vi "WILT Step 6.vi"(7 "Station Number in":u32, 8 "Error In":errorcluster, 10 "Step 3 Input":T1, 11 "Dryer Step 5 In":T3 {"Night Cycle Count" format="%04d"; "Day Cycle Count" format="%04d"}) -> (0 "Error Out":errorcluster, 2 "Step 5 Output":T1, 3 "Dryer Step 5 Output":T3 {"Night Cycle Count" format="%04d"; "Day Cycle Count" format="%04d"})   [LabVIEW 2016]
uses:
  Type Definitions/WILT Station Test State Cluster.ctl
  Type Definitions/WILT Dryer Test State.ctl
  Type Definitions/WILT Dryer.ctl
  Type Definitions/WILT Dryer Details.ctl
  Type Definitions/WILT Agilent Channel Definition.ctl
  Type Definitions/WILT DAQ Data.ctl
  Globals/WILT Globals Main Program.vi
panel:
  # "Day"
  # "Night"
  # "Day"
  # "Night"
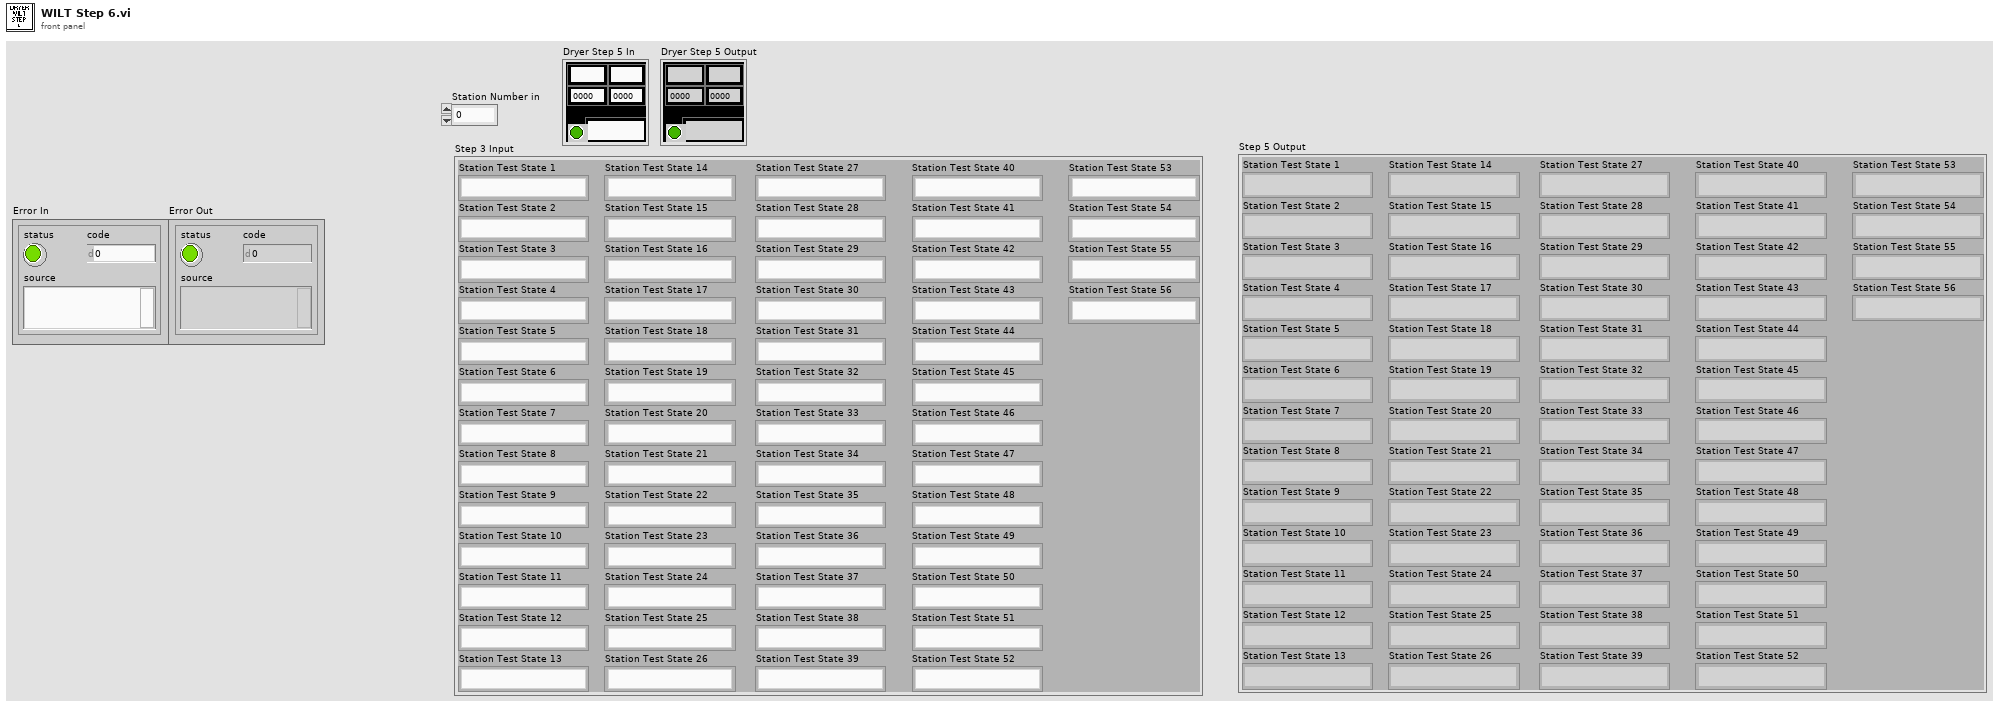
[diagram p1: front panel]
types:
  T1 = typedef "WILT Station Test State Cluster.ctl" = cluster{"Station Test State 1":T2, "Station Test State 2":T2, "Station Test State 3":T2, "Station Test State 4":T2, "Station Test State 5":T2, "Station Test State 6":T2, "Station Test State 7":T2, "Station Test State 8":T2, "Station Test State 9":T2, "Station Test State 10":T2, "Station Test State 11":T2, "Station Test State 12":T2, "Station Test State 13":T2, "Station Test State 14":T2, "Station Test State 15":T2, "Station Test State 16":T2, "Station Test State 17":T2, "Station Test State 18":T2, "Station Test State 19":T2, "Station Test State 20":T2, "Station Test State 21":T2, "Station Test State 22":T2, "Station Test State 23":T2, "Station Test State 24":T2, "Station Test State 25":T2, "Station Test State 26":T2, "Station Test State 27":T2, "Station Test State 28":T2, "Station Test State 29":T2, "Station Test State 30":T2, "Station Test State 31":T2, "Station Test State 32":T2, "Station Test State 33":T2, "Station Test State 34":T2, "Station Test State 35":T2, "Station Test State 36":T2, "Station Test State 37":T2, "Station Test State 38":T2, "Station Test State 39":T2, "Station Test State 40":T2, "Station Test State 41":T2, "Station Test State 42":T2, "Station Test State 43":T2, "Station Test State 44":T2, "Station Test State 45":T2, "Station Test State 46":T2, "Station Test State 47":T2, "Station Test State 48":T2, "Station Test State 49":T2, "Station Test State 50":T2, "Station Test State 51":T2, "Station Test State 52":T2, "Station Test State 53":T2, "Station Test State 54":T2, "Station Test State 55":T2, "Station Test State 56":T2}
  T2 = typedef "WILT Dryer Test State.ctl" = enum16{"No Serial Number", "Waiting for Dryer To Start", "Drying Clothes", "Water Injection 1 (On)", "Water Injection 1 Timer", "Water Injection 1 (Off)", "Pause Dryer", "Sending Start Stop CMD", "Pause Dryer 2", "Sending Start Stop CMD 2", "Drying Clothes 2", "Water Injection 2 (On)", "Water Injection 2 Timer", "Water Injection 2 (Off)", "Drying Clothes 3", "Cooling Down", "Sending Start Stop CMD 3", "Increment Cycle"}
  T3 = typedef "WILT Dryer.ctl" = cluster{"Lab ID":string, "Day Cycle Count":i32, "Station Label":string, "Dryer Details":T4, "Status Color":u32, "Invisible Button":bool, "Night Cycle Count":i32, "Station Index":i32, "Cycle Index":string, "Audit Alert":bool, "Agilent Channel Definition":T5, "DAQ Data":T6}
  T4 = typedef "WILT Dryer Details.ctl" = cluster{"Station":string, "Lab ID":string, "TR Number":string}
  T5 = typedef "WILT Agilent Channel Definition.ctl" = cluster{"Channel":string, "Station":string, "Label":string, "Agilent Station":string, "Data":dbl}
  T6 = typedef "WILT DAQ Data.ctl" = cluster{"L1 Current":dbl, "L2 Current":dbl, "Temperature  Deg F (TC)":dbl, "Volts":dbl, "Volts (208)":dbl, "SW (208)":dbl}
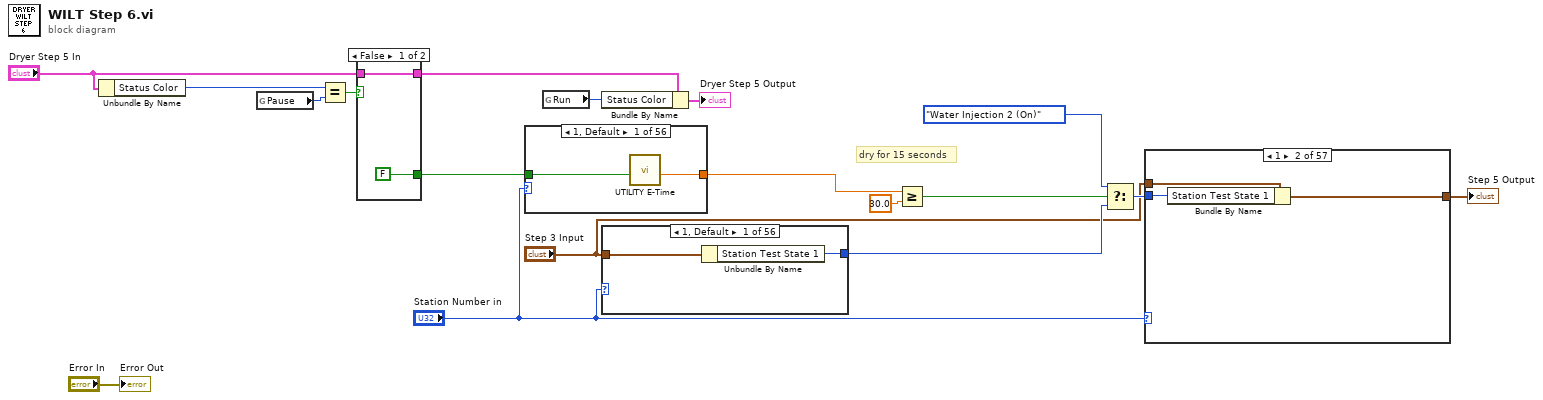
[diagram p0: block diagram]
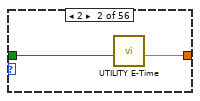
[diagram p2: hidden frame]
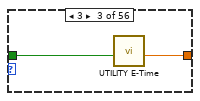
[diagram p3: hidden frame]
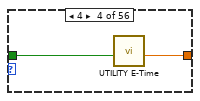
[diagram p4: hidden frame]
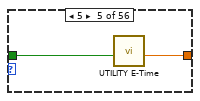
[diagram p5: hidden frame]
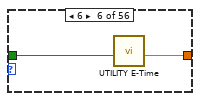
[diagram p6: hidden frame]
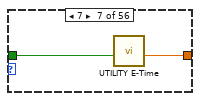
[diagram p7: hidden frame]
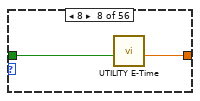
[diagram p8: hidden frame]
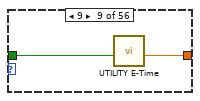
[diagram p9: hidden frame]
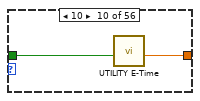
[diagram p10: hidden frame]
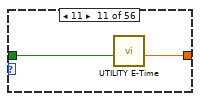
[diagram p11: hidden frame]
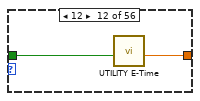
[diagram p12: hidden frame]
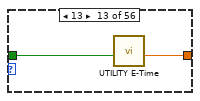
[diagram p13: hidden frame]
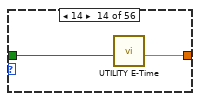
[diagram p14: hidden frame]
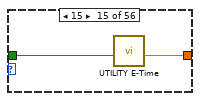
[diagram p15: hidden frame]
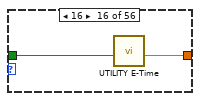
[diagram p16: hidden frame]
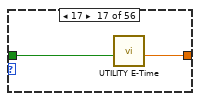
[diagram p17: hidden frame]
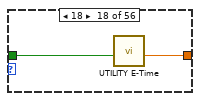
[diagram p18: hidden frame]
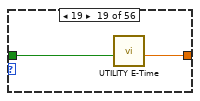
[diagram p19: hidden frame]
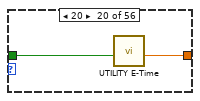
[diagram p20: hidden frame]
diagram:
  # "dry for 15 seconds"
  n1 = Unbundle By Name("Dryer Step 5 In") -> ("Status Color"=w12:u32)
  n2 = global read "WILT Globals Main Program.vi" "Pause"() -> (w4:u32)
  n3 = Equal?(x=w12, y=w4) -> (x = y?=w5:bool)
  n4 = case shown="False" w5 {
    tunnel: [FALSE TRUE] -> w2
    tunnel: "Dryer Step 5 In" -> [w19 w21]
    tunnel: [w19 w21] -> w3
    frame False {
    }
    frame True {
    }
  }
  n5 = case shown="1, Default" "Station Number in" {
    tunnel: [w24 w25 w27 w29 w31 w33 w35 w37 w39 w41 w43 w45 w47 w49 w51 w53 w55 w57 w59 w61 w63 w65 w67 w69 w71 w73 w75 w77 w79 w81 w83 w85 w87 w89 w91 w93 w95 w97 w99 w101 w103 w105 w107 w109 w111 w113 w115 w117 w119 w121 w123 w125 w127 w129 w131 w133] -> w1
    tunnel: w2 -> [w23 w26 w28 w30 w32 w34 w36 w38 w40 w42 w44 w46 w48 w50 w52 w54 w56 w58 w60 w62 w64 w66 w68 w70 w72 w74 w76 w78 w80 w82 w84 w86 w88 w90 w92 w94 w96 w98 w100 w102 w104 w106 w108 w110 w112 w114 w116 w118 w120 w122 w124 w126 w128 w130 w132 w134]
    frame 1, Default {
      n6 = call "UTILITY E-Time.vi"("Reset"=w23) -> ("Elapsed Time (sec)"=w24:dbl)  [unwired: 8 in, 2 out]
    }
    frame 2 {
      n7 = call "UTILITY E-Time.vi"("Reset"=w26) -> ("Elapsed Time (sec)"=w25:dbl)  [unwired: 8 in, 2 out]
    }
    frame 3 {
      n8 = call "UTILITY E-Time.vi"("Reset"=w28) -> ("Elapsed Time (sec)"=w27:dbl)  [unwired: 8 in, 2 out]
    }
    frame 4 {
      n9 = call "UTILITY E-Time.vi"("Reset"=w30) -> ("Elapsed Time (sec)"=w29:dbl)  [unwired: 8 in, 2 out]
    }
    frame 5 {
      n10 = call "UTILITY E-Time.vi"("Reset"=w32) -> ("Elapsed Time (sec)"=w31:dbl)  [unwired: 8 in, 2 out]
    }
    frame 6 {
      n11 = call "UTILITY E-Time.vi"("Reset"=w34) -> ("Elapsed Time (sec)"=w33:dbl)  [unwired: 8 in, 2 out]
    }
    frame 7 {
      n12 = call "UTILITY E-Time.vi"("Reset"=w36) -> ("Elapsed Time (sec)"=w35:dbl)  [unwired: 8 in, 2 out]
    }
    frame 8 {
      n13 = call "UTILITY E-Time.vi"("Reset"=w38) -> ("Elapsed Time (sec)"=w37:dbl)  [unwired: 8 in, 2 out]
    }
    frame 9 {
      n14 = call "UTILITY E-Time.vi"("Reset"=w40) -> ("Elapsed Time (sec)"=w39:dbl)  [unwired: 8 in, 2 out]
    }
    frame 10 {
      n15 = call "UTILITY E-Time.vi"("Reset"=w42) -> ("Elapsed Time (sec)"=w41:dbl)  [unwired: 8 in, 2 out]
    }
    frame 11 {
      n16 = call "UTILITY E-Time.vi"("Reset"=w44) -> ("Elapsed Time (sec)"=w43:dbl)  [unwired: 8 in, 2 out]
    }
    frame 12 {
      n17 = call "UTILITY E-Time.vi"("Reset"=w46) -> ("Elapsed Time (sec)"=w45:dbl)  [unwired: 8 in, 2 out]
    }
    frame 13 {
      n18 = call "UTILITY E-Time.vi"("Reset"=w48) -> ("Elapsed Time (sec)"=w47:dbl)  [unwired: 8 in, 2 out]
    }
    frame 14 {
      n19 = call "UTILITY E-Time.vi"("Reset"=w50) -> ("Elapsed Time (sec)"=w49:dbl)  [unwired: 8 in, 2 out]
    }
    frame 15 {
      n20 = call "UTILITY E-Time.vi"("Reset"=w52) -> ("Elapsed Time (sec)"=w51:dbl)  [unwired: 8 in, 2 out]
    }
    frame 16 {
      n21 = call "UTILITY E-Time.vi"("Reset"=w54) -> ("Elapsed Time (sec)"=w53:dbl)  [unwired: 8 in, 2 out]
    }
    frame 17 {
      n22 = call "UTILITY E-Time.vi"("Reset"=w56) -> ("Elapsed Time (sec)"=w55:dbl)  [unwired: 8 in, 2 out]
    }
    frame 18 {
      n23 = call "UTILITY E-Time.vi"("Reset"=w58) -> ("Elapsed Time (sec)"=w57:dbl)  [unwired: 8 in, 2 out]
    }
    frame 19 {
      n24 = call "UTILITY E-Time.vi"("Reset"=w60) -> ("Elapsed Time (sec)"=w59:dbl)  [unwired: 8 in, 2 out]
    }
    frame 20 {
      n25 = call "UTILITY E-Time.vi"("Reset"=w62) -> ("Elapsed Time (sec)"=w61:dbl)  [unwired: 8 in, 2 out]
    }
    frame 21 {
      n26 = call "UTILITY E-Time.vi"("Reset"=w64) -> ("Elapsed Time (sec)"=w63:dbl)  [unwired: 8 in, 2 out]
    }
    frame 22 {
      n27 = call "UTILITY E-Time.vi"("Reset"=w66) -> ("Elapsed Time (sec)"=w65:dbl)  [unwired: 8 in, 2 out]
    }
    frame 23 {
      n28 = call "UTILITY E-Time.vi"("Reset"=w68) -> ("Elapsed Time (sec)"=w67:dbl)  [unwired: 8 in, 2 out]
    }
    frame 24 {
      n29 = call "UTILITY E-Time.vi"("Reset"=w70) -> ("Elapsed Time (sec)"=w69:dbl)  [unwired: 8 in, 2 out]
    }
    frame 25 {
      n30 = call "UTILITY E-Time.vi"("Reset"=w72) -> ("Elapsed Time (sec)"=w71:dbl)  [unwired: 8 in, 2 out]
    }
    frame 26 {
      n31 = call "UTILITY E-Time.vi"("Reset"=w74) -> ("Elapsed Time (sec)"=w73:dbl)  [unwired: 8 in, 2 out]
    }
    frame 27 {
      n32 = call "UTILITY E-Time.vi"("Reset"=w76) -> ("Elapsed Time (sec)"=w75:dbl)  [unwired: 8 in, 2 out]
    }
    frame 28 {
      n33 = call "UTILITY E-Time.vi"("Reset"=w78) -> ("Elapsed Time (sec)"=w77:dbl)  [unwired: 8 in, 2 out]
    }
    frame 29 {
      n34 = call "UTILITY E-Time.vi"("Reset"=w80) -> ("Elapsed Time (sec)"=w79:dbl)  [unwired: 8 in, 2 out]
    }
    frame 30 {
      n35 = call "UTILITY E-Time.vi"("Reset"=w82) -> ("Elapsed Time (sec)"=w81:dbl)  [unwired: 8 in, 2 out]
    }
    frame 31 {
      n36 = call "UTILITY E-Time.vi"("Reset"=w84) -> ("Elapsed Time (sec)"=w83:dbl)  [unwired: 8 in, 2 out]
    }
    frame 32 {
      n37 = call "UTILITY E-Time.vi"("Reset"=w86) -> ("Elapsed Time (sec)"=w85:dbl)  [unwired: 8 in, 2 out]
    }
    frame 33 {
      n38 = call "UTILITY E-Time.vi"("Reset"=w88) -> ("Elapsed Time (sec)"=w87:dbl)  [unwired: 8 in, 2 out]
    }
    frame 34 {
      n39 = call "UTILITY E-Time.vi"("Reset"=w90) -> ("Elapsed Time (sec)"=w89:dbl)  [unwired: 8 in, 2 out]
    }
    frame 35 {
      n40 = call "UTILITY E-Time.vi"("Reset"=w92) -> ("Elapsed Time (sec)"=w91:dbl)  [unwired: 8 in, 2 out]
    }
    frame 36 {
      n41 = call "UTILITY E-Time.vi"("Reset"=w94) -> ("Elapsed Time (sec)"=w93:dbl)  [unwired: 8 in, 2 out]
    }
    frame 37 {
      n42 = call "UTILITY E-Time.vi"("Reset"=w96) -> ("Elapsed Time (sec)"=w95:dbl)  [unwired: 8 in, 2 out]
    }
    frame 38 {
      n43 = call "UTILITY E-Time.vi"("Reset"=w98) -> ("Elapsed Time (sec)"=w97:dbl)  [unwired: 8 in, 2 out]
    }
    frame 39 {
      n44 = call "UTILITY E-Time.vi"("Reset"=w100) -> ("Elapsed Time (sec)"=w99:dbl)  [unwired: 8 in, 2 out]
    }
    frame 40 {
      n45 = call "UTILITY E-Time.vi"("Reset"=w102) -> ("Elapsed Time (sec)"=w101:dbl)  [unwired: 8 in, 2 out]
    }
    frame 41 {
      n46 = call "UTILITY E-Time.vi"("Reset"=w104) -> ("Elapsed Time (sec)"=w103:dbl)  [unwired: 8 in, 2 out]
    }
    frame 42 {
      n47 = call "UTILITY E-Time.vi"("Reset"=w106) -> ("Elapsed Time (sec)"=w105:dbl)  [unwired: 8 in, 2 out]
    }
    frame 43 {
      n48 = call "UTILITY E-Time.vi"("Reset"=w108) -> ("Elapsed Time (sec)"=w107:dbl)  [unwired: 8 in, 2 out]
    }
    frame 44 {
      n49 = call "UTILITY E-Time.vi"("Reset"=w110) -> ("Elapsed Time (sec)"=w109:dbl)  [unwired: 8 in, 2 out]
    }
    frame 45 {
      n50 = call "UTILITY E-Time.vi"("Reset"=w112) -> ("Elapsed Time (sec)"=w111:dbl)  [unwired: 8 in, 2 out]
    }
    frame 46 {
      n51 = call "UTILITY E-Time.vi"("Reset"=w114) -> ("Elapsed Time (sec)"=w113:dbl)  [unwired: 8 in, 2 out]
    }
    frame 47 {
      n52 = call "UTILITY E-Time.vi"("Reset"=w116) -> ("Elapsed Time (sec)"=w115:dbl)  [unwired: 8 in, 2 out]
    }
    frame 48 {
      n53 = call "UTILITY E-Time.vi"("Reset"=w118) -> ("Elapsed Time (sec)"=w117:dbl)  [unwired: 8 in, 2 out]
    }
    frame 49 {
      n54 = call "UTILITY E-Time.vi"("Reset"=w120) -> ("Elapsed Time (sec)"=w119:dbl)  [unwired: 8 in, 2 out]
    }
    frame 50 {
      n55 = call "UTILITY E-Time.vi"("Reset"=w122) -> ("Elapsed Time (sec)"=w121:dbl)  [unwired: 8 in, 2 out]
    }
    frame 51 {
      n56 = call "UTILITY E-Time.vi"("Reset"=w124) -> ("Elapsed Time (sec)"=w123:dbl)  [unwired: 8 in, 2 out]
    }
    frame 52 {
      n57 = call "UTILITY E-Time.vi"("Reset"=w126) -> ("Elapsed Time (sec)"=w125:dbl)  [unwired: 8 in, 2 out]
    }
    frame 53 {
      n58 = call "UTILITY E-Time.vi"("Reset"=w128) -> ("Elapsed Time (sec)"=w127:dbl)  [unwired: 8 in, 2 out]
    }
    frame 54 {
      n59 = call "UTILITY E-Time.vi"("Reset"=w130) -> ("Elapsed Time (sec)"=w129:dbl)  [unwired: 8 in, 2 out]
    }
    frame 55 {
      n60 = call "UTILITY E-Time.vi"("Reset"=w132) -> ("Elapsed Time (sec)"=w131:dbl)  [unwired: 8 in, 2 out]
    }
    frame 56 {
      n61 = call "UTILITY E-Time.vi"("Reset"=w134) -> ("Elapsed Time (sec)"=w133:dbl)  [unwired: 8 in, 2 out]
    }
  }
  n62 = global read "WILT Globals Main Program.vi" "Run"() -> (w6:u32)
  n63 = Bundle By Name(cluster=w3, "Status Color"=w6) -> (→"Dryer Step 5 Output":T3)
  n64 = case shown="1, Default" "Station Number in" {
    tunnel: "Step 3 Input" -> [w136 w138 w140 w142 w144 w146 w148 w150 w152 w154 w156 w158 w160 w162 w164 w166 w168 w170 w172 w174 w176 w178 w180 w182 w184 w186 w188 w190 w192 w194 w196 w198 w200 w202 w204 w206 w208 w210 w212 w214 w216 w218 w220 w222 w224 w226 w228 w230 w232 w234 w236 w238 w240 w242 w244 w246]
    tunnel: [w135 w137 w139 w141 w143 w145 w147 w149 w151 w153 w155 w157 w159 w161 w163 w165 w167 w169 w171 w173 w175 w177 w179 w181 w183 w185 w187 w189 w191 w193 w195 w197 w199 w201 w203 w205 w207 w209 w211 w213 w215 w217 w219 w221 w223 w225 w227 w229 w231 w233 w235 w237 w239 w241 w243 w245] -> w17
    frame 1, Default {
      n65 = Unbundle By Name(w136) -> ("Station Test State 1"=w135:T2)
    }
    frame 2 {
      n66 = Unbundle By Name(w138) -> ("Station Test State 2"=w137:T2)
    }
    frame 3 {
      n67 = Unbundle By Name(w140) -> ("Station Test State 3"=w139:T2)
    }
    frame 4 {
      n68 = Unbundle By Name(w142) -> ("Station Test State 4"=w141:T2)
    }
    frame 5 {
      n69 = Unbundle By Name(w144) -> ("Station Test State 5"=w143:T2)
    }
    frame 6 {
      n70 = Unbundle By Name(w146) -> ("Station Test State 6"=w145:T2)
    }
    frame 7 {
      n71 = Unbundle By Name(w148) -> ("Station Test State 7"=w147:T2)
    }
    frame 8 {
      n72 = Unbundle By Name(w150) -> ("Station Test State 8"=w149:T2)
    }
    frame 9 {
      n73 = Unbundle By Name(w152) -> ("Station Test State 9"=w151:T2)
    }
    frame 10 {
      n74 = Unbundle By Name(w154) -> ("Station Test State 10"=w153:T2)
    }
    frame 11 {
      n75 = Unbundle By Name(w156) -> ("Station Test State 11"=w155:T2)
    }
    frame 12 {
      n76 = Unbundle By Name(w158) -> ("Station Test State 12"=w157:T2)
    }
    frame 13 {
      n77 = Unbundle By Name(w160) -> ("Station Test State 13"=w159:T2)
    }
    frame 14 {
      n78 = Unbundle By Name(w162) -> ("Station Test State 14"=w161:T2)
    }
    frame 15 {
      n79 = Unbundle By Name(w164) -> ("Station Test State 15"=w163:T2)
    }
    frame 16 {
      n80 = Unbundle By Name(w166) -> ("Station Test State 16"=w165:T2)
    }
    frame 17 {
      n81 = Unbundle By Name(w168) -> ("Station Test State 17"=w167:T2)
    }
    frame 18 {
      n82 = Unbundle By Name(w170) -> ("Station Test State 18"=w169:T2)
    }
    frame 19 {
      n83 = Unbundle By Name(w172) -> ("Station Test State 19"=w171:T2)
    }
    frame 20 {
      n84 = Unbundle By Name(w174) -> ("Station Test State 20"=w173:T2)
    }
    frame 21 {
      n85 = Unbundle By Name(w176) -> ("Station Test State 21"=w175:T2)
    }
    frame 22 {
      n86 = Unbundle By Name(w178) -> ("Station Test State 22"=w177:T2)
    }
    frame 23 {
      n87 = Unbundle By Name(w180) -> ("Station Test State 23"=w179:T2)
    }
    frame 24 {
      n88 = Unbundle By Name(w182) -> ("Station Test State 24"=w181:T2)
    }
    frame 25 {
      n89 = Unbundle By Name(w184) -> ("Station Test State 25"=w183:T2)
    }
    frame 26 {
      n90 = Unbundle By Name(w186) -> ("Station Test State 26"=w185:T2)
    }
    frame 27 {
      n91 = Unbundle By Name(w188) -> ("Station Test State 27"=w187:T2)
    }
    frame 28 {
      n92 = Unbundle By Name(w190) -> ("Station Test State 28"=w189:T2)
    }
    frame 29 {
      n93 = Unbundle By Name(w192) -> ("Station Test State 29"=w191:T2)
    }
    frame 30 {
      n94 = Unbundle By Name(w194) -> ("Station Test State 30"=w193:T2)
    }
    frame 31 {
      n95 = Unbundle By Name(w196) -> ("Station Test State 31"=w195:T2)
    }
    frame 32 {
      n96 = Unbundle By Name(w198) -> ("Station Test State 32"=w197:T2)
    }
    frame 33 {
      n97 = Unbundle By Name(w200) -> ("Station Test State 33"=w199:T2)
    }
    frame 34 {
      n98 = Unbundle By Name(w202) -> ("Station Test State 34"=w201:T2)
    }
    frame 35 {
      n99 = Unbundle By Name(w204) -> ("Station Test State 35"=w203:T2)
    }
    frame 36 {
      n100 = Unbundle By Name(w206) -> ("Station Test State 36"=w205:T2)
    }
    frame 37 {
      n101 = Unbundle By Name(w208) -> ("Station Test State 37"=w207:T2)
    }
    frame 38 {
      n102 = Unbundle By Name(w210) -> ("Station Test State 38"=w209:T2)
    }
    frame 39 {
      n103 = Unbundle By Name(w212) -> ("Station Test State 39"=w211:T2)
    }
    frame 40 {
      n104 = Unbundle By Name(w214) -> ("Station Test State 40"=w213:T2)
    }
    frame 41 {
      n105 = Unbundle By Name(w216) -> ("Station Test State 41"=w215:T2)
    }
    frame 42 {
      n106 = Unbundle By Name(w218) -> ("Station Test State 42"=w217:T2)
    }
    frame 43 {
      n107 = Unbundle By Name(w220) -> ("Station Test State 43"=w219:T2)
    }
    frame 44 {
      n108 = Unbundle By Name(w222) -> ("Station Test State 44"=w221:T2)
    }
    frame 45 {
      n109 = Unbundle By Name(w224) -> ("Station Test State 45"=w223:T2)
    }
    frame 46 {
      n110 = Unbundle By Name(w226) -> ("Station Test State 46"=w225:T2)
    }
    frame 47 {
      n111 = Unbundle By Name(w228) -> ("Station Test State 47"=w227:T2)
    }
    frame 48 {
      n112 = Unbundle By Name(w230) -> ("Station Test State 48"=w229:T2)
    }
    frame 49 {
      n113 = Unbundle By Name(w232) -> ("Station Test State 49"=w231:T2)
    }
    frame 50 {
      n114 = Unbundle By Name(w234) -> ("Station Test State 50"=w233:T2)
    }
    frame 51 {
      n115 = Unbundle By Name(w236) -> ("Station Test State 51"=w235:T2)
    }
    frame 52 {
      n116 = Unbundle By Name(w238) -> ("Station Test State 52"=w237:T2)
    }
    frame 53 {
      n117 = Unbundle By Name(w240) -> ("Station Test State 53"=w239:T2)
    }
    frame 54 {
      n118 = Unbundle By Name(w242) -> ("Station Test State 54"=w241:T2)
    }
    frame 55 {
      n119 = Unbundle By Name(w244) -> ("Station Test State 55"=w243:T2)
    }
    frame 56 {
      n120 = Unbundle By Name(w246) -> ("Station Test State 56"=w245:T2)
    }
  }
  n121 = Greater Or Equal?(x=w1, y=30.0) -> (x >= y?=w14:bool)
  n122 = Select(t=WILT_Dryer_Test_State."Water Injection 2 (On)" ("Current State 2"), s=w14, f=w17) -> (s? t:f=w18:T2)
  n123 = case shown="1" "Station Number in" {
    tunnel: "Step 3 Input" -> [w247 w250 w253 w256 w259 w262 w265 w268 w271 w274 w277 w280 w283 w286 w289 w292 w295 w298 w301 w304 w307 w310 w313 w316 w319 w322 w325 w328 w331 w334 w337 w340 w343 w346 w349 w352 w355 w358 w361 w364 w367 w370 w373 w376 w379 w382 w385 w388 w391 w394 w397 w400 w403 w406 w409 w412 w415]
    tunnel: w18 -> [_ w249 w251 w254 w257 w260 w263 w266 w269 w272 w275 w278 w281 w284 w287 w290 w293 w296 w299 w302 w305 w308 w311 w314 w317 w320 w323 w326 w329 w332 w335 w338 w341 w344 w347 w350 w353 w356 w359 w362 w365 w368 w371 w374 w377 w380 w383 w386 w389 w392 w395 w398 w401 w404 w407 w410 w413]
    tunnel: [w247 w248 w252 w255 w258 w261 w264 w267 w270 w273 w276 w279 w282 w285 w288 w291 w294 w297 w300 w303 w306 w309 w312 w315 w318 w321 w324 w327 w330 w333 w336 w339 w342 w345 w348 w351 w354 w357 w360 w363 w366 w369 w372 w375 w378 w381 w384 w387 w390 w393 w396 w399 w402 w405 w408 w411 w414] -> w15
    frame 0, Default {
      # "Not a valid station. Do nothing"
    }
    frame 1 {
      n124 = Bundle By Name(cluster=w250, "Station Test State 1"=w249) -> (w248:T1)
    }
    frame 2 {
      n125 = Bundle By Name(cluster=w253, "Station Test State 2"=w251) -> (w252:T1)
    }
    frame 3 {
      n126 = Bundle By Name(cluster=w256, "Station Test State 3"=w254) -> (w255:T1)
    }
    frame 4 {
      n127 = Bundle By Name(cluster=w259, "Station Test State 4"=w257) -> (w258:T1)
    }
    frame 5 {
      n128 = Bundle By Name(cluster=w262, "Station Test State 5"=w260) -> (w261:T1)
    }
    frame 6 {
      n129 = Bundle By Name(cluster=w265, "Station Test State 6"=w263) -> (w264:T1)
    }
    frame 7 {
      n130 = Bundle By Name(cluster=w268, "Station Test State 7"=w266) -> (w267:T1)
    }
    frame 8 {
      n131 = Bundle By Name(cluster=w271, "Station Test State 8"=w269) -> (w270:T1)
    }
    frame 9 {
      n132 = Bundle By Name(cluster=w274, "Station Test State 9"=w272) -> (w273:T1)
    }
    frame 10 {
      n133 = Bundle By Name(cluster=w277, "Station Test State 10"=w275) -> (w276:T1)
    }
    frame 11 {
      n134 = Bundle By Name(cluster=w280, "Station Test State 11"=w278) -> (w279:T1)
    }
    frame 12 {
      n135 = Bundle By Name(cluster=w283, "Station Test State 12"=w281) -> (w282:T1)
    }
    frame 13 {
      n136 = Bundle By Name(cluster=w286, "Station Test State 13"=w284) -> (w285:T1)
    }
    frame 14 {
      n137 = Bundle By Name(cluster=w289, "Station Test State 14"=w287) -> (w288:T1)
    }
    frame 15 {
      n138 = Bundle By Name(cluster=w292, "Station Test State 15"=w290) -> (w291:T1)
    }
    frame 16 {
      n139 = Bundle By Name(cluster=w295, "Station Test State 16"=w293) -> (w294:T1)
    }
    frame 17 {
      n140 = Bundle By Name(cluster=w298, "Station Test State 17"=w296) -> (w297:T1)
    }
    frame 18 {
      n141 = Bundle By Name(cluster=w301, "Station Test State 18"=w299) -> (w300:T1)
    }
    frame 19 {
      n142 = Bundle By Name(cluster=w304, "Station Test State 19"=w302) -> (w303:T1)
    }
    frame 20 {
      n143 = Bundle By Name(cluster=w307, "Station Test State 20"=w305) -> (w306:T1)
    }
    frame 21 {
      n144 = Bundle By Name(cluster=w310, "Station Test State 21"=w308) -> (w309:T1)
    }
    frame 22 {
      n145 = Bundle By Name(cluster=w313, "Station Test State 22"=w311) -> (w312:T1)
    }
    frame 23 {
      n146 = Bundle By Name(cluster=w316, "Station Test State 23"=w314) -> (w315:T1)
    }
    frame 24 {
      n147 = Bundle By Name(cluster=w319, "Station Test State 24"=w317) -> (w318:T1)
    }
    frame 25 {
      n148 = Bundle By Name(cluster=w322, "Station Test State 25"=w320) -> (w321:T1)
    }
    frame 26 {
      n149 = Bundle By Name(cluster=w325, "Station Test State 26"=w323) -> (w324:T1)
    }
    frame 27 {
      n150 = Bundle By Name(cluster=w328, "Station Test State 27"=w326) -> (w327:T1)
    }
    frame 28 {
      n151 = Bundle By Name(cluster=w331, "Station Test State 28"=w329) -> (w330:T1)
    }
    frame 29 {
      n152 = Bundle By Name(cluster=w334, "Station Test State 29"=w332) -> (w333:T1)
    }
    frame 30 {
      n153 = Bundle By Name(cluster=w337, "Station Test State 30"=w335) -> (w336:T1)
    }
    frame 31 {
      n154 = Bundle By Name(cluster=w340, "Station Test State 31"=w338) -> (w339:T1)
    }
    frame 32 {
      n155 = Bundle By Name(cluster=w343, "Station Test State 32"=w341) -> (w342:T1)
    }
    frame 33 {
      n156 = Bundle By Name(cluster=w346, "Station Test State 33"=w344) -> (w345:T1)
    }
    frame 34 {
      n157 = Bundle By Name(cluster=w349, "Station Test State 34"=w347) -> (w348:T1)
    }
    frame 35 {
      n158 = Bundle By Name(cluster=w352, "Station Test State 35"=w350) -> (w351:T1)
    }
    frame 36 {
      n159 = Bundle By Name(cluster=w355, "Station Test State 36"=w353) -> (w354:T1)
    }
    frame 37 {
      n160 = Bundle By Name(cluster=w358, "Station Test State 37"=w356) -> (w357:T1)
    }
    frame 38 {
      n161 = Bundle By Name(cluster=w361, "Station Test State 38"=w359) -> (w360:T1)
    }
    frame 39 {
      n162 = Bundle By Name(cluster=w364, "Station Test State 39"=w362) -> (w363:T1)
    }
    frame 40 {
      n163 = Bundle By Name(cluster=w367, "Station Test State 40"=w365) -> (w366:T1)
    }
    frame 41 {
      n164 = Bundle By Name(cluster=w370, "Station Test State 41"=w368) -> (w369:T1)
    }
    frame 42 {
      n165 = Bundle By Name(cluster=w373, "Station Test State 42"=w371) -> (w372:T1)
    }
    frame 43 {
      n166 = Bundle By Name(cluster=w376, "Station Test State 43"=w374) -> (w375:T1)
    }
    frame 44 {
      n167 = Bundle By Name(cluster=w379, "Station Test State 44"=w377) -> (w378:T1)
    }
    frame 45 {
      n168 = Bundle By Name(cluster=w382, "Station Test State 45"=w380) -> (w381:T1)
    }
    frame 46 {
      n169 = Bundle By Name(cluster=w385, "Station Test State 46"=w383) -> (w384:T1)
    }
    frame 47 {
      n170 = Bundle By Name(cluster=w388, "Station Test State 47"=w386) -> (w387:T1)
    }
    frame 48 {
      n171 = Bundle By Name(cluster=w391, "Station Test State 48"=w389) -> (w390:T1)
    }
    frame 49 {
      n172 = Bundle By Name(cluster=w394, "Station Test State 49"=w392) -> (w393:T1)
    }
    frame 50 {
      n173 = Bundle By Name(cluster=w397, "Station Test State 50"=w395) -> (w396:T1)
    }
    frame 51 {
      n174 = Bundle By Name(cluster=w400, "Station Test State 51"=w398) -> (w399:T1)
    }
    frame 52 {
      n175 = Bundle By Name(cluster=w403, "Station Test State 52"=w401) -> (w402:T1)
    }
    frame 53 {
      n176 = Bundle By Name(cluster=w406, "Station Test State 53"=w404) -> (w405:T1)
    }
    frame 54 {
      n177 = Bundle By Name(cluster=w409, "Station Test State 54"=w407) -> (w408:T1)
    }
    frame 55 {
      n178 = Bundle By Name(cluster=w412, "Station Test State 55"=w410) -> (w411:T1)
    }
    frame 56 {
      n179 = Bundle By Name(cluster=w415, "Station Test State 56"=w413) -> (w414:T1)
    }
  }
  "Step 5 Output" <- w15
  "Error Out" <- "Error In"
